vi "Dashboard Main.vi"() -> ()   [LabVIEW 2011]
uses:
  <vilib>/Math Plots/2D Math Plots/2D Compass/2D Compass XCtrl/2D Compass.xctl
  2_17_2012-Robot-Code/Dashboard Datatype.ctl
  <vilib>/Rock Robotics/WPI/DriverStation/WPI_DriverStationDigitalData.ctl
  <vilib>/Math Plots/2D Math Plots/2D Compass/2D Compass Datatype/Public/Plot Helper (Vector).vi
  <vilib>/Math Plots/2D Math Plots/2D Compass/2D Compass Datatype/2D Compass Datatype.lvclass
panel:
  out "Status":T1(ring)
  out "Hammer Lower Limit":bool
  out "Hammer Upper Limit":bool
  out "Angle Reset":bool
  out "Ball Detector":bool
  out "Robot IP Address":string="10.0.0.2"
  out "Elevator Speed":dbl(slide) scale=-1.0..1.0
  out "Collector Speed":dbl(slide) scale=-1.0..1.0
  out "Right Speed":dbl(slide) scale=-1.0..1.0
  out "Left Speed":dbl(slide) scale=-1.0..1.0
  in  "Video Enable":bool=TRUE
  out "Camera Image":T2(plugin-control)
  out "Camera IP Address":string
  in  "Suggest":bool=TRUE
  out "Shooter Angle":refnum<class "2D Plot Datatype.lvclass">[](xcontrol) caption="2D Compass"
  out "Dashboard Datatype Warning":string="Warning: The Dashboard Datatype used by the robot project and this dashboard do not match.\nSee diagram for more details."
  out "Image Error Message":string="Timeout in Camera Communications"
  # "Shooter Angle"
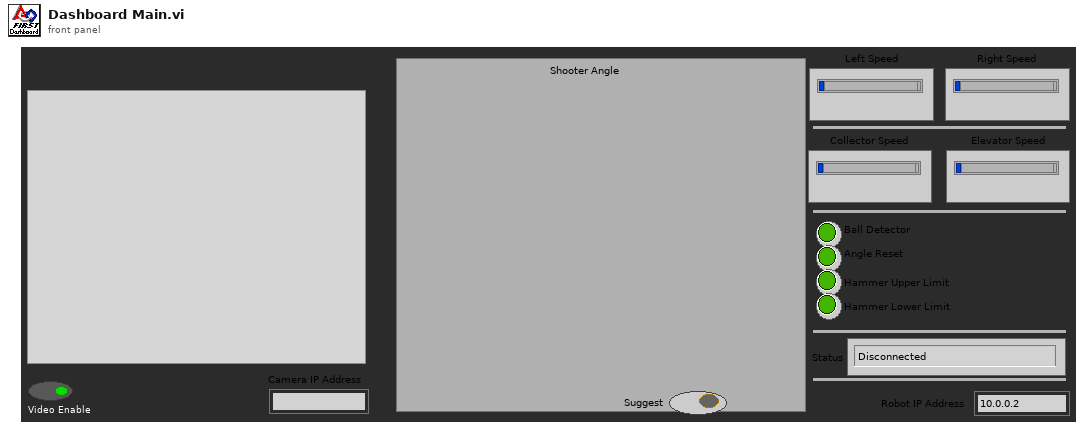
[diagram p1: front panel]
types:
  T1 = enum8{"Disconnected", "E-Stop", "Disabled", "Enabled"}
  T2 = typedef "IMAQ Image.ctl" = refnum<image>
  T3 = typedef "Dashboard Datatype.ctl" = cluster{cluster{"AnalogModule[0]":cluster{"Channel[0]":sgl, "Channel[1]":sgl, "Channel[2]":sgl, "Channel[3]":sgl, "Channel[4]":sgl, "Channel[5]":sgl, "Channel[6]":sgl, "Channel[7]":sgl}, "AnalogModule[1]":cluster{"Channel[0]":sgl, "Channel[1]":sgl, "Channel[2]":sgl, "Channel[3]":sgl, "Channel[4]":sgl, "Channel[5]":sgl, "Channel[6]":sgl, "Channel[7]":sgl}}, cluster{"DigitalModule[0]":T4, "DigitalModule[1]":T4}, "Solenoid":u8, "Shooting":dbl, "Shooting Speed":dbl, "Distance":dbl, "Left Speed":dbl, "Right Speed ":dbl, "Collector Speed ":dbl, "Elevator Speed ":dbl}
  T4 = typedef "WPI_DriverStationDigitalData.ctl" = cluster{"Relay Fwd":u8, "Relay Rev":u8, "GPIO":u16, "GPIO_OE":u16, "PWM":cluster{"PWM[0]":u8, "PWM[1]":u8, "PWM[2]":u8, "PWM[3]":u8, "PWM[4]":u8, "PWM[5]":u8, "PWM[6]":u8, "PWM[7]":u8, "PWM[8]":u8, "PWM[9]":u8}}
  T5 = typedef "Image Type" = u32
  T6 = cluster{cluster{"AnalogModule[0]":cluster{"Channel[0]":sgl, "Channel[1]":sgl, "Channel[2]":sgl, "Channel[3]":sgl, "Channel[4]":sgl, "Channel[5]":sgl, "Channel[6]":sgl, "Channel[7]":sgl}, "AnalogModule[1]":cluster{"Channel[0]":sgl, "Channel[1]":sgl, "Channel[2]":sgl, "Channel[3]":sgl, "Channel[4]":sgl, "Channel[5]":sgl, "Channel[6]":sgl, "Channel[7]":sgl}}, cluster{"DigitalModule[0]":T4, "DigitalModule[1]":T4}, "Solenoid":u8}
  T7 = typedef "LVRectTypeDef.ctl" = cluster{"left":i16, "top":i16, "right":i16, "bottom":i16}
  T8 = cluster{"Competition mode":bool, "Robot Link":bool, "Autonomous":bool, "Enabled":bool, "E-Stop":bool}
  T9 = cluster{"AnalogModule[0]":cluster{"Channel[0]":sgl, "Channel[1]":sgl, "Channel[2]":sgl, "Channel[3]":sgl, "Channel[4]":sgl, "Channel[5]":sgl, "Channel[6]":sgl, "Channel[7]":sgl}, "AnalogModule[1]":cluster{"Channel[0]":sgl, "Channel[1]":sgl, "Channel[2]":sgl, "Channel[3]":sgl, "Channel[4]":sgl, "Channel[5]":sgl, "Channel[6]":sgl, "Channel[7]":sgl}}
  T10 = cluster{"DigitalModule[0]":T4, "DigitalModule[1]":T4}
  T11 = cluster{"Channel[0]":sgl, "Channel[1]":sgl, "Channel[2]":sgl, "Channel[3]":sgl, "Channel[4]":sgl, "Channel[5]":sgl, "Channel[6]":sgl, "Channel[7]":sgl}[]
  T12 = cluster{"Channel[0]":sgl, "Channel[1]":sgl, "Channel[2]":sgl, "Channel[3]":sgl, "Channel[4]":sgl, "Channel[5]":sgl, "Channel[6]":sgl, "Channel[7]":sgl}
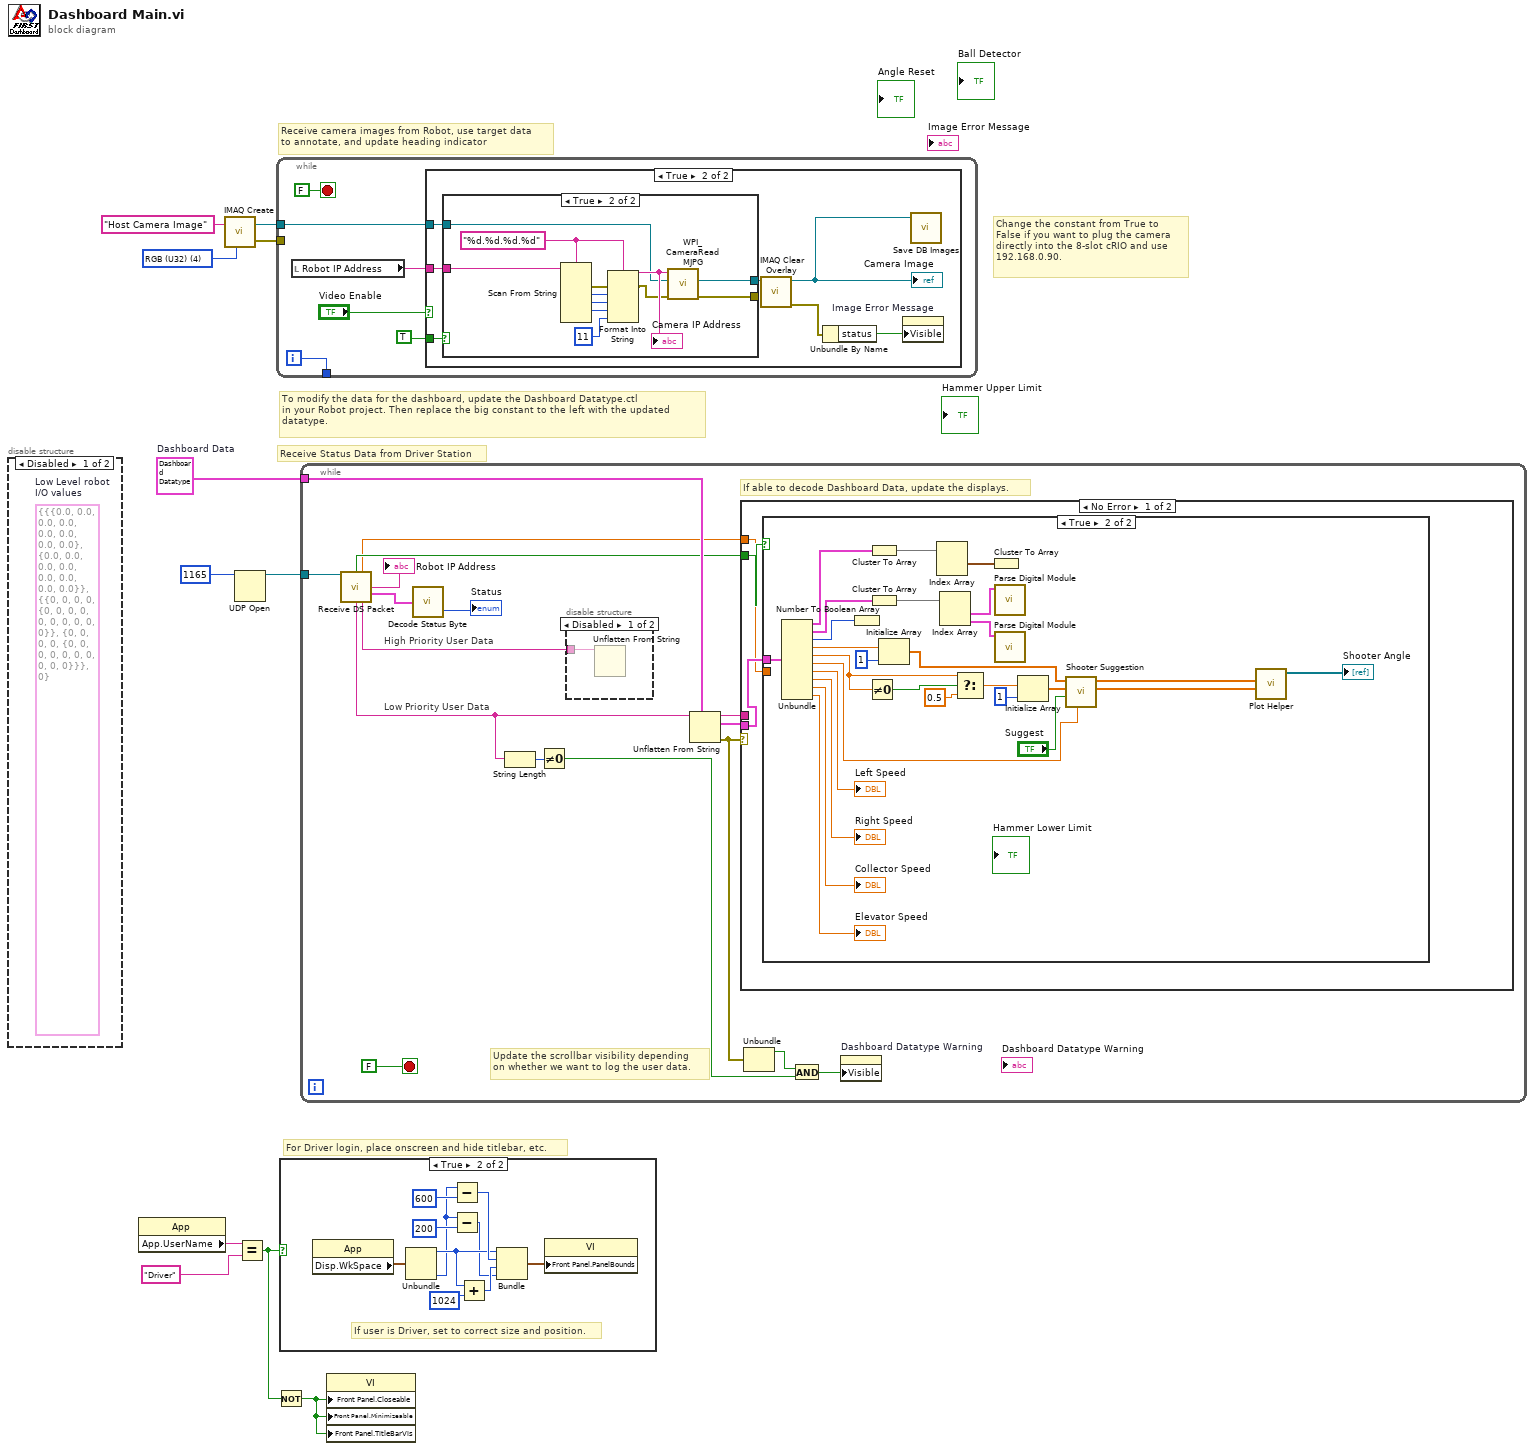
[diagram p0: block diagram]
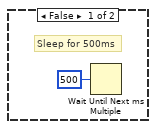
[diagram p7: hidden frame]
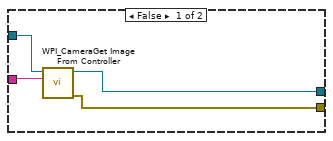
[diagram p8: hidden frame]
diagram:
  w1 = T3 {{"AnalogModule[0]"={"Channel[0]"=0.0, "Channel[1]"=0.0, "Channel[2]"=0.0, "Channel[3]"=0.0, "Channel[4]"=0.0, "Channel[5]"=0.0, "Channel[6]"=0.0, "Channel[7]"=0.0}, "AnalogModule[1]"={"Channel[0]"=0.0, "Channel[1]"=0.0, "Channel[2]"=0.0, "Channel[3]"=0.0, "Channel[4]"=0.0, "Channel[5]"=0.0, "Channel[6]"=0.0, "Channel[7]"=0.0}}, {"DigitalModule[0]"={"Relay Fwd"=0, "Relay Rev"=0, "GPIO"=0, "GPIO_OE"=0, "PWM"={"PWM[0]"=0, "PWM[1]"=0, "PWM[2]"=0, "PWM[3]"=0, "PWM[4]"=0, "PWM[5]"=0, "PWM[6]"=0, "PWM[7]"=0, "PWM[8]"=0, "PWM[9]"=0}}, "DigitalModule[1]"={"Relay Fwd"=0, "Relay Rev"=0, "GPIO"=0, "GPIO_OE"=0, "PWM"={"PWM[0]"=0, "PWM[1]"=0, "PWM[2]"=0, "PWM[3]"=0, "PWM[4]"=0, "PWM[5]"=0, "PWM[6]"=0, "PWM[7]"=0, "PWM[8]"=0, "PWM[9]"=0}}}, "Solenoid"=0, "Shooting"=0.0, "Shooting Speed"=0.0, "Distance"=0.0, "Left Speed"=0.0, "Right Speed "=0.0, "Collector Speed "=0.0, "Elevator Speed "=0.0}  # Dashboard Data
  w9 = T5 4 items=["Grayscale (U8)", "Grayscale (I16)", "Grayscale (SGL)", "Complex (CSG)", "RGB (U32)", "HSL (U32)", "RGB (U64)"] ("Image Type")
  # "Change the constant from True to\nFalse if you want to plug the camera\ndirectly into the 8-slot cRIO and use\n192.168.0.90."
  # "For Driver login, place onscreen and hide titlebar, etc."
  # "To modify the data for the dashboard, update the Dashboard Datatype.ctl\nin your Robot project. Then replace the big constant to the left with the updated\ndatatype."
  # "Receive Status Data from Driver Station"
  # "Receive camera images from Robot, use target data\nto annotate, and update heading indicator"
  n1 = disable-structure shown="Disabled" {
    frame Disabled {
      (unwired) T6 {{"AnalogModule[0]"={"Channel[0]"=0.0, "Channel[1]"=0.0, "Channel[2]"=0.0, "Channel[3]"=0.0, "Channel[4]"=0.0, "Channel[5]"=0.0, "Channel[6]"=0.0, "Channel[7]"=0.0}, "AnalogModule[1]"={"Channel[0]"=0.0, "Channel[1]"=0.0, "Channel[2]"=0.0, "Channel[3]"=0.0, "Channel[4]"=0.0, "Channel[5]"=0.0, "Channel[6]"=0.0, "Channel[7]"=0.0}}, {"DigitalModule[0]"={"Relay Fwd"=0, "Relay Rev"=0, "GPIO"=0, "GPIO_OE"=0, "PWM"={"PWM[0]"=0, "PWM[1]"=0, "PWM[2]"=0, "PWM[3]"=0, "PWM[4]"=0, "PWM[5]"=0, "PWM[6]"=0, "PWM[7]"=0, "PWM[8]"=0, "PWM[9]"=0}}, "DigitalModule[1]"={"Relay Fwd"=0, "Relay Rev"=0, "GPIO"=0, "GPIO_OE"=0, "PWM"={"PWM[0]"=0, "PWM[1]"=0, "PWM[2]"=0, "PWM[3]"=0, "PWM[4]"=0, "PWM[5]"=0, "PWM[6]"=0, "PWM[7]"=0, "PWM[8]"=0, "PWM[9]"=0}}}, "Solenoid"=0}  # Low Level robot I/O values
    }
    frame Enabled {
    }
  }
  n2 = property class="App"() -> ("App.UserName"=w4:string)  [unwired: 2 in, 2 out]
  n3 = call "IMAQ Create"("Image Name"="Host Camera Image", "Image Type"=w9) -> ("New Image"=w7:T2, "error out"=w6:errorcluster)  [unwired: 2 in, 1 out]
  n4 = UDP Open(11:u16 1165 ("port")) -> (port=w10:refnum<k16>)  [unwired: 2 in, 4 out]
  n5 = Equal?(x=w4, y="Driver") -> (x = y?=w3:bool)
  n6 = Not(x=w3) -> (.not. x?=w2:bool)
  n7 = while {
    tunnel: w7 -> [w15]
    tunnel: w6 -> [_]
    tunnel: [w12] -> _
    i -> [w12]
    stop <- FALSE stop-if-true
    n8 = local read "Robot IP Address"() -> (w16:string)
    n9 = case shown="True" "Video Enable" {
      tunnel: w16 -> [_ w25]
      tunnel: w15 -> [_ w24]
      tunnel: TRUE -> [_ w19]
      frame False {
        # "Sleep for 500ms"
        n10 = Wait Until Next ms Multiple(millisecond multiple=u32 500) -> ()  [unwired: 1 out]
      }
      frame True {
        n11 = case shown="True" w19 {
          tunnel: w24 -> [w28 w35]
          tunnel: [w26 w33] -> _
          tunnel: [w27 w34] -> w21
          tunnel: w25 -> [w29 w38]
          frame False {
            n12 = call <vilib>:"WPI_CameraGet Image From Controller.vi"("Controller Address"=w29, "Image"=w28) -> ("error out"=w26:errorcluster, "Image Out"=w27:T2)  [unwired: 2 in, 6 out]
          }
          frame True {
            w30 = "%d.%d.%d.%d" ("format string")
            n13 = Scan From String(format string=w30, input string=w38) -> (error out=w37:errorcluster, output 1=w39:i32, output 2=w40:i32, output 3=w41:i32)  [unwired: 2 in, 7 out]
            n14 = Format Into String(format string=w30, error in=w37, w39, w40, w41, 11 ("IP Suffix:")) -> (resulting string=w36:string, error out=w32:errorcluster)  [unwired: 1 in]
            "Camera IP Address" <- w36
            n15 = call <vilib>:"WPI_CameraRead MJPG.vi"("error in"=w32, "Image"=w35, "address"=w36) -> ("error out"=w33:errorcluster, "Image Out"=w34:T2)  [unwired: 7 in]
          }
        }
        n16 = call "IMAQ Clear Overlay"("Image"=w21) -> ("error out"=w22:errorcluster, "Image Out"=w20:T2)  [unwired: 2 in, 7 out]
        "Camera Image" <- w20
        n17 = Unbundle By Name(w22) -> ("status"=w23:bool)
        n18 = property on="Image Error Message" class="Str"("Visible"=w23) -> ()  [unwired: 2 in, 2 out]
        n19 = call "Save DB Images.vi"("Image"=w20) -> ()  [unwired: 2 in, 1 out]
      }
    }
  }
  n20 = case shown="True" w3 {
    frame False {
    }
    frame True {
      # "If user is Driver, set to correct size and position."
      n21 = property class="App"() -> ("Disp.WkSpace"=w51:T7)  [unwired: 2 in, 2 out]
      n22 = Unbundle(w51) -> ("left"=w46:i16, "bottom"=w42:i16)  [unwired: 2 out]
      n23 = Subtract(x=w42, y=600) -> (x-y=w48:i32)
      n24 = Subtract(x=w42, y=200) -> (x-y=w43:i32)
      n25 = Add(x=w46, y=1024) -> (x+y=w47:i32)
      n26 = Bundle("left"=w46, w48, w47, w43) -> (w50:cluster{"left":i16, i32, i32, i32})  [unwired: 1 out]
      n27 = property class="VI"("Front Panel.PanelBounds"=w50) -> ()  [unwired: 2 in, 2 out]
    }
  }
  n28 = while {
    tunnel: w10 -> [w66]
    tunnel: w1 -> [w65]
    stop <- FALSE stop-if-true
    # "High Priority User Data"
    # "Low Priority User Data"
    # "Update the scrollbar visibility depending\non whether we want to log the user data."
    # "If able to decode Dashboard Data, update the displays."
    n29 = call "Receive DS Packet.vi"("Recv Socket"=w66) -> ("New Dashboard Data"=w62:bool, "Battery"=w54:sgl, "Robot IP Address"=→"Robot IP Address":string, "Status"=w67:T8, "Low Priority User Data"=w56:string, "High Priority User Data"=w55:string)  [unwired: 1 in, 8 out]
    n30 = call "Decode Status Byte.vi"("Status Byte"=w67) -> ("Status"=→"Status":T1)  [unwired: 1 out]
    n31 = String Length(string=w56) -> (length=w57:i32)
    n32 = Not Equal To 0?(x=w57) -> (x != 0?=w60:bool)
    n33 = disable-structure shown="Disabled" {
      disable-tunnel: w55 -> [w69 _]
      frame Disabled {
        n34 = Unflatten From String(binary string=w69) -> ()  [unwired: 2 in, 5 out]
      }
      frame Enabled {
      }
    }
    n35 = Unflatten From String(type=w65, binary string=w56) -> (rest of the binary string=w58:string, value=w64:T3, error out=w63:errorcluster)  [unwired: 1 in, 2 out]
    n36 = case shown="No Error" w63 {
      tunnel: w64 -> [w72 _]
      tunnel: w62 -> [w71 _]
      tunnel: w58 -> [_ _]
      tunnel: w54 -> [w70 _]
      frame No Error {
        n37 = case shown="True" w71 {
          tunnel: w72 -> [_ w95]
          tunnel: w70 -> [_ _]
          frame False {
            # "Don't update if the robot hasn't sent new data"
          }
          frame True {
            n38 = Unbundle(w95) -> (w92:T9, w93:T10, "Solenoid"=w94:u8, "Shooting"=w78:dbl, "Shooting Speed"=w86:dbl, "Distance"=w77:dbl, "Left Speed"=→"Left Speed":dbl, "Right Speed"=→"Right Speed":dbl, "Collector Speed"=→"Collector Speed":dbl, "Elevator Speed"=→"Elevator Speed":dbl)
            n39 = Number To Boolean Array(number=w94) -> ()  [unwired: 1 out]
            n40 = Not Equal To 0?(x=w86) -> (x != 0?=w87:bool)
            n41 = Cluster To Array(cluster=w92) -> (array=w99:T11)
            n42 = Cluster To Array(cluster=w93) -> (array=w98:T4[])
            n43 = Initialize Array(w78, 1 ("dimension size")) -> (w82:dbl[])
            n44 = Index Array(array=w99) -> (element #1=w91:T12)  [unwired: 2 in, 1 out]
            n45 = Index Array(array=w98) -> (element #1=w97:T4, element #2=w96:T4)  [unwired: 2 in]
            n46 = Select(t=w86, s=w87, f=0.5) -> (s? t:f=w84:dbl)
            n47 = Cluster To Array(cluster=w91) -> ()  [unwired: 1 out]
            n48 = call "Parse Digital Module.vi"("DigitalModule"=w97) -> ()  [unwired: 11 out]
            n49 = call "Parse Digital Module.vi"("DigitalModule"=w96) -> ()  [unwired: 11 out]
            n50 = Initialize Array(w84, 1 ("dimension size")) -> (w80:dbl[])
            n51 = call "Shooter Suggestion.vi"("Distance"=w77, "Suggest"="Suggest", "Radius in"=w80, "Theta in"=w82) -> ("Radius out"=w79:dbl[], "Theta Out"=w81:dbl[])  [unwired: 6 in]
            n52 = call-poly <vilib>:"Plot Helper.vi"("radius vector"=w79, "theta vector"=w81) -> ("2D Plot Class Obj Array out"=→"Shooter Angle":refnum<class "2D Plot Datatype.lvclass">[])  [unwired: 2 in, 7 out]
          }
        }
      }
      frame Error {
        # "Your datatypes don't match. The Dashboard Datatype.ctl in your Robot project\nand the big constant to the left of the loop need to match."
      }
    }
    n53 = Unbundle(w63) -> ("status"=w59:bool)  [unwired: 2 out]
    n54 = And(x=w59, y=w60) -> (x .and. y?=w61:bool)
    n55 = property on="Dashboard Datatype Warning" class="Str"("Visible"=w61) -> ()  [unwired: 2 in, 2 out]
  }
  n56 = property class="VI"("Front Panel.Closeable"=w2, "Front Panel.Minimizeable"=w2, "Front Panel.TitleBarVis"=w2) -> ()  [unwired: 2 in, 2 out]
